vi "Check for Cooler State Changes.vi"(4 "error in (no error)":errorcluster, 7 "State Machine Data":T1) -> (0 "error out":errorcluster, 3 "Cooler Need Adjusting?":bool)   [LabVIEW 2015, in "Startup Processes.lvlib"]
uses:
  Startup Processes.lvlib
  _typedefs/State Machine Conditions.ctl
  _typedefs/Machine Modes.ctl
  _typedefs/Subpanel Names.ctl
  Config Data/Config Data.lvclass
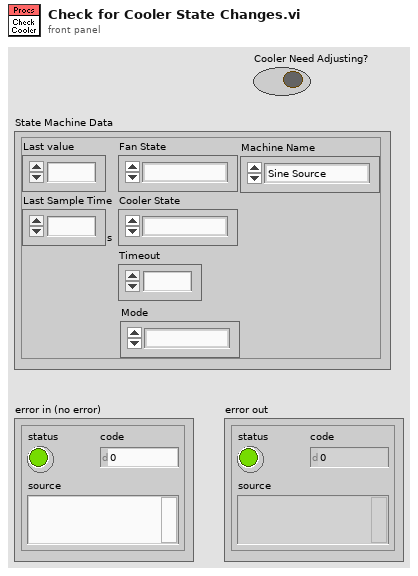
[diagram p1: front panel]
types:
  T1 = typedef "Startup Processes.lvlib/State Machine Conditions.ctl" = cluster{"Last value":dbl, "Last Sample Time":dbl[unit], "Fan State":enum16{"Off", "On"}, "Cooler State":enum16{"Off", "On"}, "Timeout":i32, "Mode":T2, "Machine Name":T3}
  T2 = typedef "Startup Processes.lvlib/Machine Modes.ctl" = enum16{"Startup", "Run"}
  T3 = typedef "Startup Processes.lvlib/Subpanel Names.ctl" = enum16{"Sine Source", "Ramp Source", "Hen House TC", "Dog House TC", "Out House TC"}
  T4 = cluster{"Error High Level":dbl, "Warning High Level":dbl, "Warning Low Level":dbl, "Error Low Level":dbl, "Sample Interval":dbl[unit]}
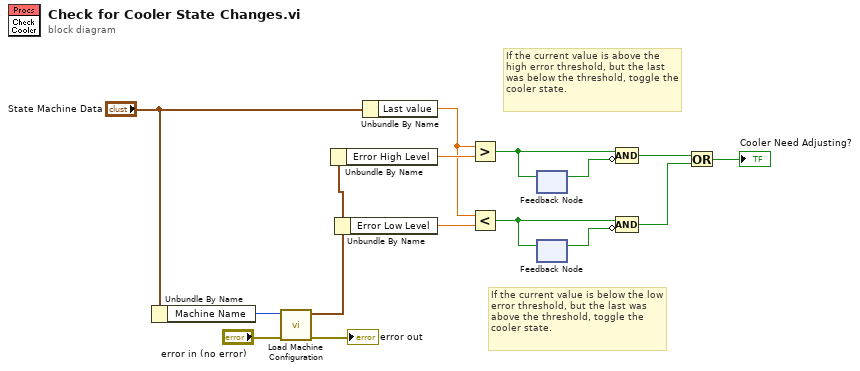
[diagram p0: block diagram]
diagram:
  # "If the current value is below the low error threshold, but the last was above the threshold, toggle the cooler state."
  # "If the current value is above the high error threshold, but the last was below the threshold, toggle the cooler state."
  n1 = Unbundle By Name("State Machine Data") -> ("Machine Name"=w4:T3)
  n2 = call "Load Machine Configuration.vi"("error in (no error)"="error in (no error)", "Instance Name"=w4) -> ("error out"=→"error out":errorcluster, "TC Parameters"=w1:T4)  [unwired: 4 in]
  n3 = Unbundle By Name(w1) -> ("Error High Level"=w8:dbl)
  n4 = Unbundle By Name(w1) -> ("Error Low Level"=w7:dbl)
  n5 = Unbundle By Name("State Machine Data") -> ("Last value"=w6:dbl)
  n6 = Greater?(x=w6, y=w8) -> (0:w15:bool)
  n7 = Less?(x=w6, y=w7) -> (x < y?=w12:bool)
  n8 = feedback #1() -> (w14:bool)  [unwired: 1 in]
  n9 = feedback-in #1(w15) -> ()
  n10 = feedback #2() -> (w13:bool)  [unwired: 1 in]
  n11 = feedback-in #2(w12) -> ()
  n12 = Compound Arithmetic op=AND(w15, invert w14) -> (w11:bool)
  n13 = Compound Arithmetic op=AND(w12, invert w13) -> (w10:bool)
  n14 = Or(x=w11, y=w10) -> (x .or. y?=→"Cooler Need Adjusting?":bool)
